vi "Build Convolution Support v2.vi"(3 "X Array 2":dbl[](array[numeric]), 5 "X Array 1":dbl[](array[numeric])) -> (1 "X Arrays Convolution Support":dbl[](array[numeric]))   [LabVIEW 2021, in "Fits.lvlib"]
uses:
  Fits.lvlib
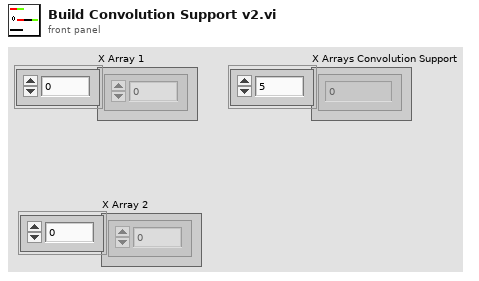
[diagram p1: front panel]
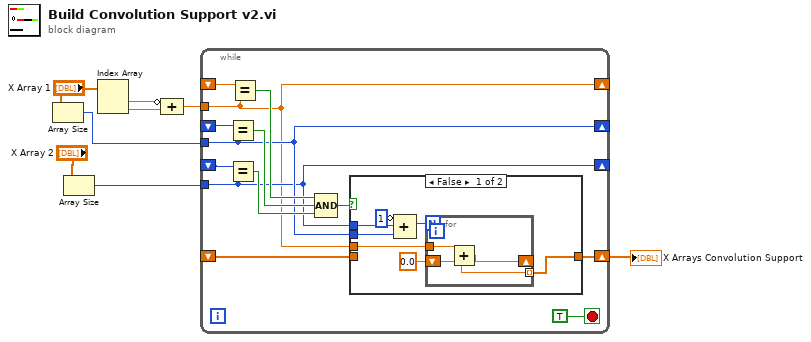
[diagram p0: block diagram]
diagram:
  n1 = Array Size(array="X Array 1") -> (size(s)=w3:i32)
  n2 = Array Size(array="X Array 2") -> (size(s)=w2:i32)
  n3 = Index Array(array="X Array 1") -> (element #1=w6:dbl, element #2=w5:dbl)  [unwired: 2 in]
  n4 = Compound Arithmetic op=ADD(invert w6, w5) -> (w4:dbl)
  n5 = while {
    shift-right: [w9] -> _
    shift-left: _ -> [w21]
    tunnel: w4 -> [w9]
    tunnel: w3 -> [w11]
    shift-right: [w11] -> _
    shift-left: _ -> [w20]
    tunnel: w2 -> [w10]
    shift-right: [w10] -> _
    shift-left: _ -> [w19]
    shift-right: [w12] -> w1
    shift-left: _ -> [w13]
    stop <- TRUE stop-if-true
    n6 = Equal?(x=w20, y=w11) -> (x = y?=w17:bool)
    n7 = Equal?(x=w19, y=w10) -> (x = y?=w16:bool)
    n8 = Equal?(x=w21, y=w9) -> (x = y?=w18:bool)
    n9 = Compound Arithmetic op=AND(w18, w17, w16) -> (w15:bool)
    n10 = case shown="False" w15 {
      tunnel: w13 -> [_ w32]
      tunnel: [w22 w32] -> w12
      tunnel: w11 -> [w27 _]
      tunnel: w10 -> [w28 _]
      tunnel: w9 -> [w24 _]
      frame False {
        n11 = Compound Arithmetic op=ADD(invert 1 ("value"), w28, w27) -> (w25:i32)
        n12 = for {
          N: w25 -> [_]
          tunnel: w24 -> [w31]
          shift-right: [w30] -> _
          shift-left: 0.0 -> [w29]
          tunnel: [w29] -> w22 mode=indexing
          n13 = Add(x=w31, y=w29) -> (x+y=w30:dbl)
        }
      }
      frame True {
      }
    }
  }
  "X Arrays Convolution Support" <- w1
